vi "Choreo_EventMarker_Equals.vi"(9 "OtherChoreoEvent":T1, 11 "ChoreoEvent":T1) -> (3 "Equal":bool)   [LabVIEW 2019, in "ChoreoLib.lvlib"]
doc: "Check to see if two event markers are equal\n\nInputs:\n -- EventMarker - cluster - The event marker data cluster \n -- OtherEventMarker - cluster - The other event marker data cluster to check\n\nOutputs: \n -- equal - boolean - TRUE if event markers are equal"
uses:
  ChoreoLib.lvlib
  TypeDef/ChoreoEventMarker.ctl
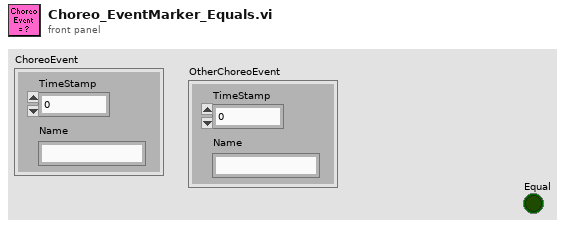
[diagram p1: front panel]
types:
  T1 = typedef "ChoreoLib.lvlib/ChoreoEventMarker.ctl" = cluster{"TimeStamp":dbl, "Name":string}
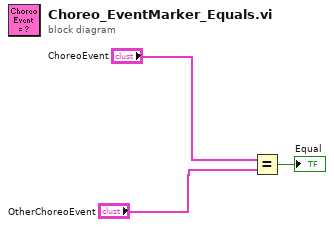
[diagram p0: block diagram]
diagram:
  n1 = Equal?(x="ChoreoEvent", y="OtherChoreoEvent") -> (x = y?=→"Equal":bool)
